vi "Graphs.vi"() -> ()   [LabVIEW 2018]
uses:
  <vilib>/Instr/_visa.llb/VISA Configure Serial Port (Instr).vi
panel:
  out "output cluster":T1
  in  "stop":bool
  out "Temp":dynamicdata(graph)
  out "Hum":dynamicdata(graph)
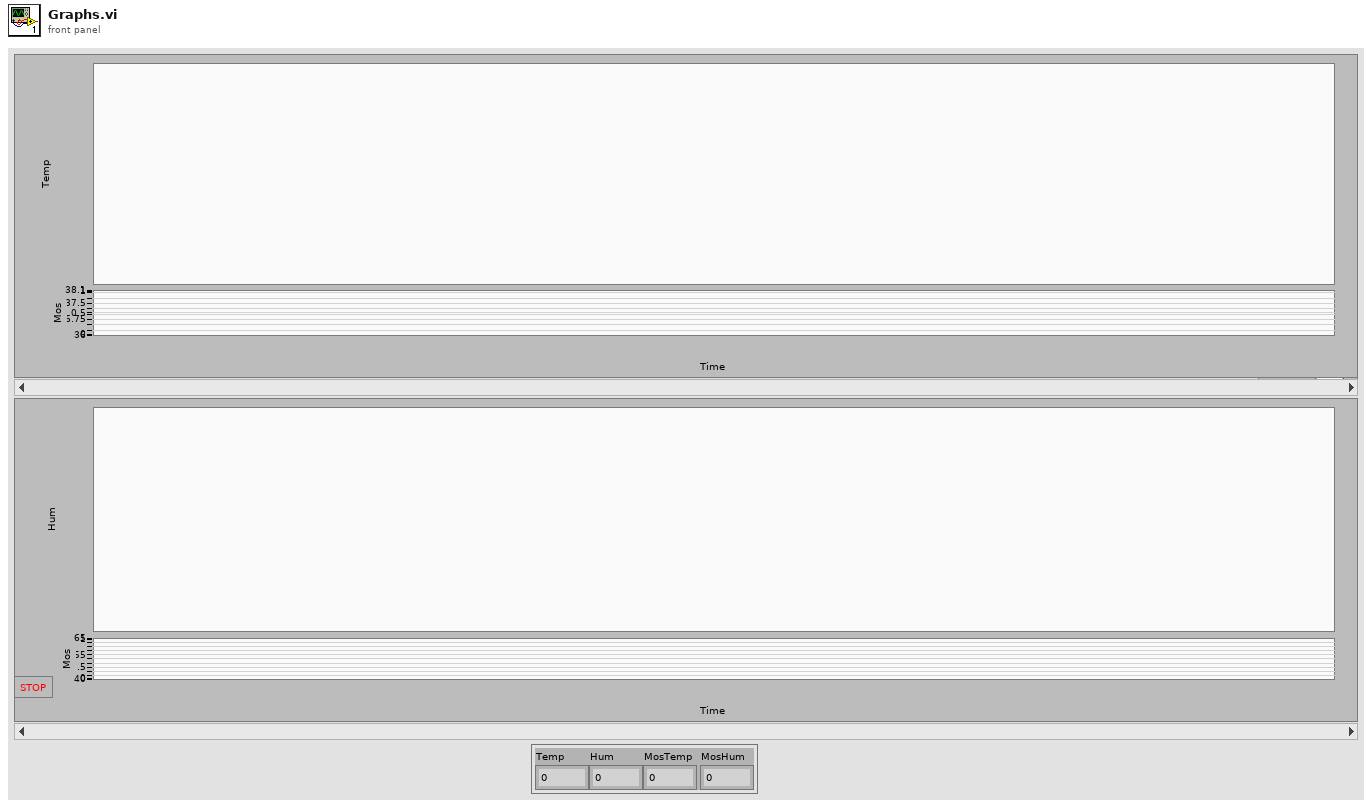
[diagram p1: front panel]
types:
  T1 = cluster{"Temp":dbl, "Hum":dbl, "MosTemp":dbl, "MosHum":dbl}
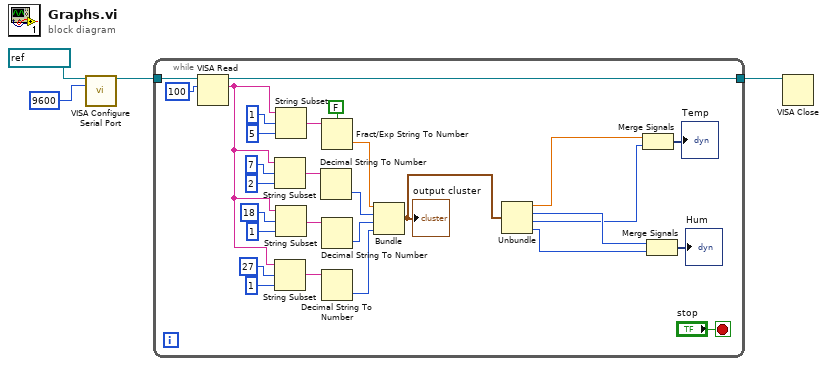
[diagram p0: block diagram]
diagram:
  n1 = call-poly "VISA Configure Serial Port"("VISA resource name"=refnum<visa-resource-name> "COM4", "baud rate (9600)"=u32 9600) -> ("VISA resource name out"=w2:refnum<visa-resource-name>)  [unwired: 12 in, 1 out]
  n2 = while {
    tunnel: w2 -> [w32]
    tunnel: [w33] -> w3
    stop <- "stop" stop-if-true
    n3 = VISA Read(VISA resource name=w32, byte count=u32 100) -> (VISA resource name out=w33:refnum<visa-resource-name>, read buffer=w19:string)  [unwired: 1 in, 2 out]
    n4 = String Subset(string=w19, offset (0)=7, length (rest)=2 ("length (rest)")) -> (substring=w18:string)
    n5 = String Subset(string=w19, offset (0)=27, length (rest)=1 ("length (rest)")) -> (substring=w17:string)
    n6 = String Subset(string=w19, offset (0)=1, length (rest)=5 ("length (rest)")) -> (substring=w28:string)
    n7 = String Subset(string=w19, offset (0)=18, length (rest)=1 ("length (rest)")) -> (substring=w16:string)
    n8 = Decimal String To Number(string=w18) -> (number=w14:i32)  [unwired: 2 in, 1 out]
    n9 = Fract/Exp String To Number(use system decimal point (T)=FALSE, string=w28) -> (number=w15:dbl)  [unwired: 2 in, 1 out]
    n10 = Decimal String To Number(string=w16) -> (number=w13:i32)  [unwired: 2 in, 1 out]
    n11 = Decimal String To Number(string=w17) -> (number=w12:i32)  [unwired: 2 in, 1 out]
    n12 = Bundle(w15, w14, w13, w12) -> (w9:cluster{dbl, i32, i32, i32})  [unwired: 1 in]
    "output cluster" <- w9
    n13 = Unbundle(w9) -> (w8:dbl, w7:i32, w5:i32, w6:i32)
    n14 = Merge Signals(w8, w5) -> (→"Temp":dynamicdata)
    n15 = Merge Signals(w7, w6) -> (→"Hum":dynamicdata)
  }
  n16 = VISA Close(VISA resource name=w3) -> ()  [unwired: 1 in, 1 out]
